vi "init_motor.vi"(8 "error in":errorcluster, 9 "velocity":dbl, 10 "steps_per_rev":i32, 11 "VISA in":refnum<visa-resource-name>) -> (0 "error out":errorcluster, 1 "status":bool, 3 "VISA out":refnum<visa-resource-name>)   [LabVIEW 2019]
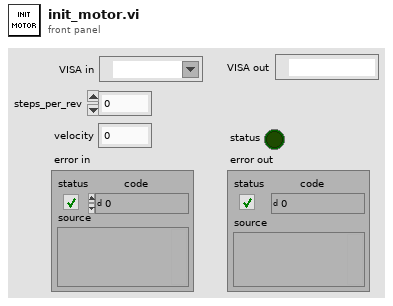
[diagram p1: front panel]
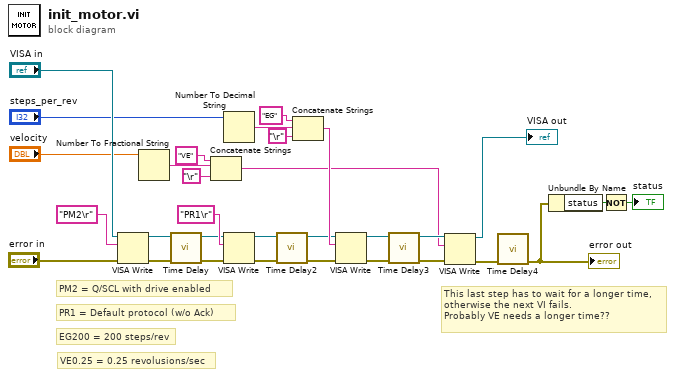
[diagram p0: block diagram]
diagram:
  # "This last step has to wait for a longer time,\notherwise the next VI fails.\nProbably VE needs a longer time??"
  # "VE0.25 = 0.25 revolusions/sec"
  # "EG200 = 200 steps/rev"
  # "PR1 = Default protocol (w/o Ack)"
  # "PM2 = Q/SCL with drive enabled"
  n1 = VISA Write(VISA resource name="VISA in", write buffer="PM2\r", error in (no error)="error in") -> (VISA resource name out=w8:refnum<visa-resource-name>, error out=w26:errorcluster)  [unwired: 1 out]
  n2 = Number To Fractional String(number="velocity") -> (F-format string=w13:string)  [unwired: 3 in]
  n3 = call "Time Delay"("error in (no error)"=w26) -> ("error out"=w11:errorcluster)  [unwired: 10 in]
  n4 = Concatenate Strings("VE", w13, "\r") -> (w4:string)
  n5 = Number To Decimal String(number="steps_per_rev") -> (decimal integer string=w20:string)  [unwired: 1 in]
  n6 = VISA Write(VISA resource name=w8, write buffer="PR1\r", error in (no error)=w11) -> (VISA resource name out=w7:refnum<visa-resource-name>, error out=w24:errorcluster)  [unwired: 1 out]
  n7 = call "Time Delay2"("error in (no error)"=w24) -> ("error out"=w10:errorcluster)  [unwired: 10 in]
  n8 = Concatenate Strings("EG", w20, "\r") -> (w17:string)
  n9 = VISA Write(VISA resource name=w7, write buffer=w17, error in (no error)=w10) -> (VISA resource name out=w6:refnum<visa-resource-name>, error out=w18:errorcluster)  [unwired: 1 out]
  n10 = call "Time Delay3"("error in (no error)"=w18) -> ("error out"=w9:errorcluster)  [unwired: 10 in]
  n11 = VISA Write(VISA resource name=w6, write buffer=w4, error in (no error)=w9) -> (VISA resource name out=→"VISA out":refnum<visa-resource-name>, error out=w12:errorcluster)  [unwired: 1 out]
  n12 = call "Time Delay4"("error in (no error)"=w12) -> ("error out"=w3:errorcluster)  [unwired: 10 in]
  "error out" <- w3
  n13 = Unbundle By Name(w3) -> ("status"=w2:bool)
  n14 = Not(x=w2) -> (.not. x?=→"status":bool)
